vi "SFC_WIPPVICheck.vi"(5 "UserNo":string, 6 "CheckRS":string, 7 "Process":string, 8 "error in (no error)":errorcluster caption="错误输入（无错误）", 9 "ProdLine":string, 10 "SID":string, 11 "Traceability 引用句柄":refnum<k24>) -> (0 "error out":errorcluster caption="错误输出", 2 "SFC_WIPPVICheck":string, 3 "Traceability 引用句柄输出":refnum<k24>)   [LabVIEW 2014, in "Traceability.lvlib"]
uses:
  D:/webservice/Traceability.dll
  Traceability.dll
  Traceability.lvlib
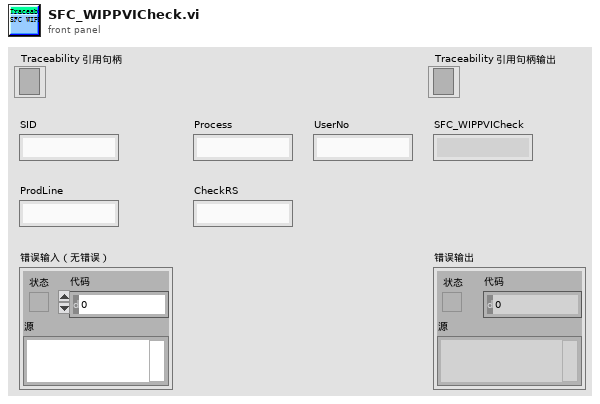
[diagram p1: front panel]
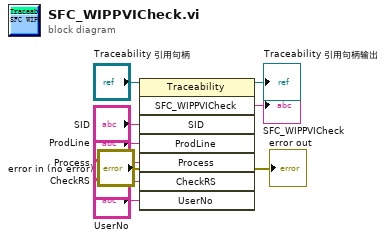
[diagram p0: block diagram]
diagram:
  n1 = invoke class="Traceability" method="SFC_WIPPVICheck"(reference="Traceability 引用句柄", error in="error in (no error)", "SID"="SID", "ProdLine"="ProdLine", "Process"="Process", "CheckRS"="CheckRS", "UserNo"="UserNo") -> (reference out=→"Traceability 引用句柄输出":refnum<k24>, error out=→"error out":errorcluster, "SFC_WIPPVICheck"=→"SFC_WIPPVICheck":string)  [unwired: 1 in, 5 out]
